vi "GT Get Task.vi"(7 "pTaskData":u32, 8 "error in (no error)":errorcluster caption="错误输入（无错误）", 9 "pTaskType":i16, 10 "taskIndex":i16, 11 "cardNum":i16) -> (0 "error out":errorcluster caption="错误输出", 1 "pTaskType out":i16, 3 "function return":i16, 5 "pTaskData out":u32)   [LabVIEW 2020, in "gts1.lvlib"]
doc: "GT_API GT_GetTask(short cardNum,short taskIndex,short *pTaskType,void *pTaskData);"
uses:
  gts1.lvlib
  dll/32bit/multi_card/gts.dll
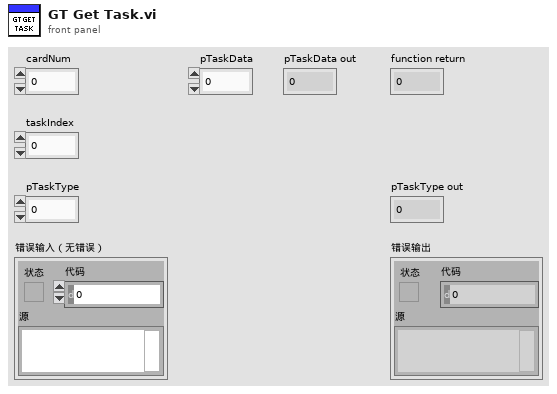
[diagram p1: front panel]
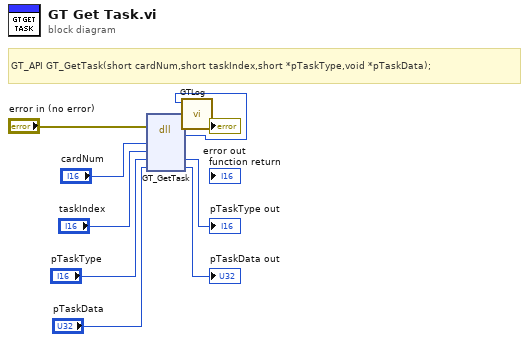
[diagram p0: block diagram]
diagram:
  # "GT_API GT_GetTask(short cardNum,short taskIndex,short *pTaskType,void *pTaskData);"
  n1 = dll-call lib="C:/1228/dll/32bit/multi_card/gts.dll" fn="GT_GetTask"(error in="error in (no error)", "cardNum"="cardNum", "taskIndex"="taskIndex", "pTaskType"="pTaskType", "pTaskData"="pTaskData") -> (error out=w3:errorcluster, w1:i16, "pTaskType"=→"pTaskType out":i16, "pTaskData"=→"pTaskData out":u32)  [unwired: 4 in, 1 out]
  n2 = call "GTLog.vi"("error in (no error)"=w3, "Numeric"=w1) -> ("error out"=→"error out":errorcluster)  [unwired: 9 in]
